vi "connect.vi"(0 "Network Manager IP Address or Hostname":string, 1 "Identity":T1 {"type" items=["Client", "Service"]}, 5 "Network Manager port":u16=1875, 9 "timeout ms":i32=10000, 11 "error in":errorcluster, 12 "username":string, 13 "password":string) -> (4 "connection ID":refnum<k5>, 6 "queue out":refnum<queue>, 15 "error out":errorcluster)   [LabVIEW 2010]
uses:
  i3-json-1.0.0-10/JSON Parsing/Get Object Parameter Files/Get Object Parameter - String.vi
  i3-json-1.0.0-10/i3-json.lvlib
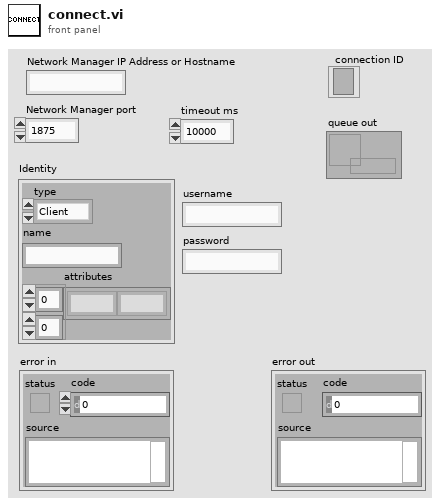
[diagram p1: front panel]
types:
  T1 = cluster{"type":u16, "name":string, "attributes":string[][]}
  T2 = enum16{"Standard", "Buffered", "CRLF", "Immediate"}
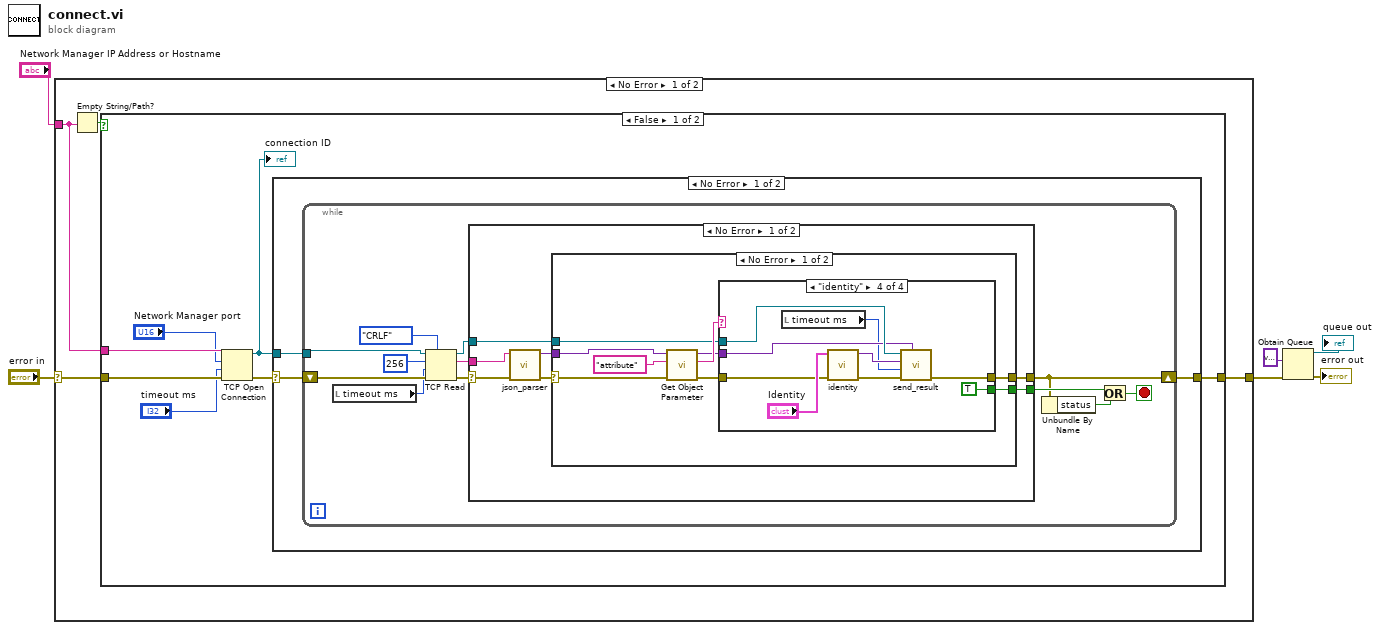
[diagram p0: block diagram]
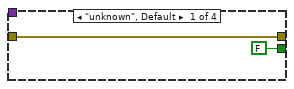
[diagram p2: hidden frame]
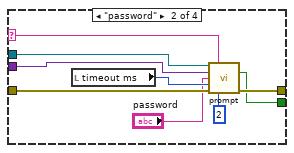
[diagram p3: hidden frame]
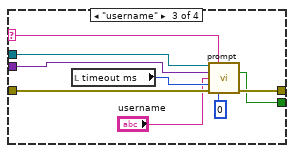
[diagram p4: hidden frame]
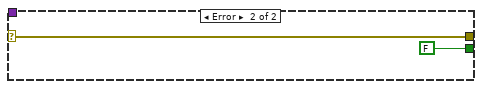
[diagram p5: hidden frame]
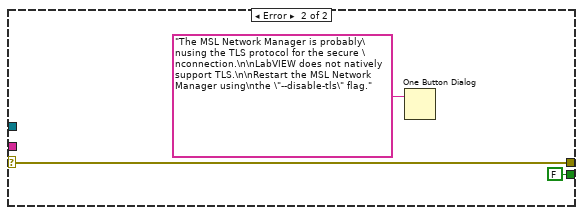
[diagram p6: hidden frame]
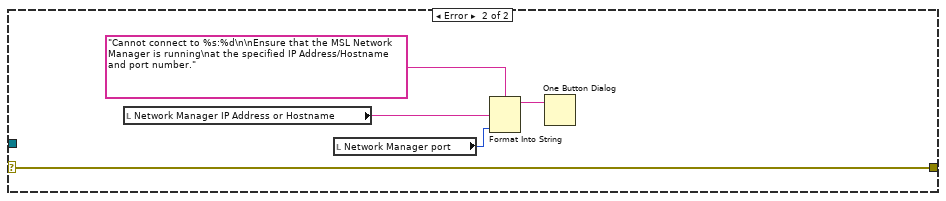
[diagram p7: hidden frame]
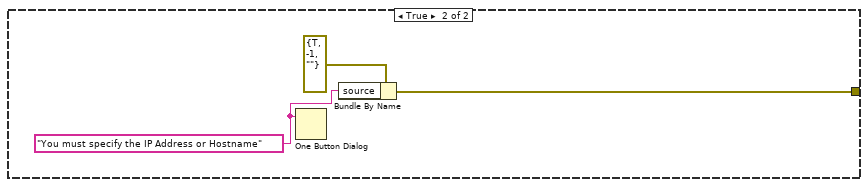
[diagram p8: hidden frame]
diagram:
  n1 = case shown="No Error" "error in" {
    selector: "error in" -> [w8 w91]
    tunnel: [w9 w91] -> w4
    tunnel: "Network Manager IP Address or Hostname" -> [w7 _]
    frame No Error {
      n2 = Empty String/Path?(string/path=w7) -> (empty?=w10:bool)
      n3 = case shown="False" w10 {
        tunnel: [w16 w88] -> w9
        tunnel: w8 -> [w15 _]
        tunnel: w7 -> [w13 _]
        frame False {
          n4 = TCP Open Connection(address=w13, remote port or service name="Network Manager port", timeout ms (60000)="timeout ms", error in (no error)=w15) -> (connection ID=w14:refnum<k5>, error out=w17:errorcluster)  [unwired: 1 in]
          "connection ID" <- w14
          n5 = case shown="No Error" w17 {
            selector: w17 -> [w20 w85]
            tunnel: [w19 w85] -> w16
            tunnel: w14 -> [w18 _]
            frame No Error {
              n6 = while {
                shift-right: [w22] -> w19
                shift-left: w20 -> [w32]
                tunnel: w18 -> [w26]
                stop <- w23 stop-if-true
                n7 = local read "timeout ms"() -> (w25:i32)
                n8 = TCP Read(connection ID=w26, bytes to read=256 ("32bit integer"), error in (no error)=w32, 7:T2."CRLF" ("mode (standard)"), 9:w25) -> (connection ID out=w27:refnum<k5>, data out=w30:string, error out=w28:errorcluster)
                n9 = case shown="No Error" w28 {
                  selector: w28 -> [w39 w81]
                  tunnel: w30 -> [w33 _]
                  tunnel: [w38 w81] -> w22
                  tunnel: w27 -> [w36 _]
                  tunnel: [w35 FALSE] -> w24
                  frame No Error {
                    n10 = call "json_parser.vi"("error in"=w39, "JSON String"=w33) -> ("error out"=w34:errorcluster, "JSON Tree Out Passthrough"=w37:variant)  [unwired: 8 in]
                    n11 = case shown="No Error" w34 {
                      selector: w34 -> [w40 w79]
                      tunnel: [w48 w79] -> w38
                      tunnel: w37 -> [w46 _]
                      tunnel: w36 -> [w43 _]
                      tunnel: [w41 FALSE] -> w35
                      frame No Error {
                        n12 = call-poly "Get Object Parameter.vi"("error in (no error)"=w40, "Parameter Name"="attribute" ("name"), "JSON Tree In (JSON Object)"=w46) -> ("error out"=w45:errorcluster, "String Value"=w44:string, "JSON Tree Out Passthrough"=w42:variant)  [unwired: 5 in, 1 out]
                        n13 = case shown="\"identity\"" w44 {
                          selector: w44 -> [_ w57 w62 _]
                          tunnel: w45 -> [w50 w54 w65 w76]
                          tunnel: [w50 w53 w64 w73] -> w48
                          tunnel: w43 -> [_ w56 w68 w75]
                          tunnel: w42 -> [_ w55 w67 w72]
                          tunnel: [FALSE w52 w63 TRUE] -> w41
                          frame "unknown", Default {
                          }
                          frame "password" {
                            n14 = local read "timeout ms"() -> (w59:i32)
                            n15 = call "prompt.vi"("connection ID"=w56, "type"=w57, "JSON Tree In (JSON Object)"=w55, "default value"="password", "timeout ms"=w59, "error in"=w54, "Display Style"=u32 2) -> ("cancelled?"=w52:bool, "error out"=w53:errorcluster)  [unwired: 6 in, 1 out]
                          }
                          frame "username" {
                            n16 = local read "timeout ms"() -> (w66:i32)
                            n17 = call "prompt.vi"("connection ID"=w68, "type"=w62, "JSON Tree In (JSON Object)"=w67, "default value"="username", "timeout ms"=w66, "error in"=w65, "Display Style"=u32 0) -> ("cancelled?"=w63:bool, "error out"=w64:errorcluster)  [unwired: 6 in, 1 out]
                          }
                          frame "identity" {
                            n18 = local read "timeout ms"() -> (w69:i32)
                            n19 = call "identity.vi"("error in"=w76, "Identity"="Identity") -> ("error out"=w74:errorcluster, "JSON Tree out (JSON Object)"=w71:variant)  [unwired: 8 in]
                            n20 = call "send_result.vi"("JSON Tree In (JSON Object)"=w72, "error in"=w74, "timeout ms"=w69, "result"=w71, "connection ID"=w75) -> ("error out"=w73:errorcluster)  [unwired: 3 in, 3 out]
                          }
                        }
                      }
                      frame Error {
                      }
                    }
                  }
                  frame Error {
                    n21 = One Button Dialog(message="The MSL Network Manager is probably\nusing the TLS protocol for the secure \nconnection.\n\nLabVIEW does not natively support TLS.\n\nRestart the MSL Network Manager using\nthe \"--disable-tls\" flag.") -> ()  [unwired: 1 in, 1 out]
                  }
                }
                n22 = Unbundle By Name(w22) -> ("status"=w21:bool)
                n23 = Or(x=w24, y=w21) -> (x .or. y?=w23:bool)
              }
            }
            frame Error {
              n24 = local read "Network Manager IP Address or Hostname"() -> (w84:string)
              n25 = local read "Network Manager port"() -> (w83:u16)
              n26 = Format Into String(format string="Cannot connect to %s:%d\n\nEnsure that the MSL Network Manager is running\nat the specified IP Address/Hostname and port number.", w84, w83) -> (resulting string=w86:string)  [unwired: 2 in, 1 out]
              n27 = One Button Dialog(message=w86) -> ()  [unwired: 1 in, 1 out]
            }
          }
        }
        frame True {
          w90 = "You must specify the IP Address or Hostname" ("error source (\" \")")
          n28 = One Button Dialog(message=w90) -> ()  [unwired: 1 in, 1 out]
          n29 = Bundle By Name(cluster=errorcluster {"status"=TRUE, "code"=-1, "source"=""} ("error out"), "source"=w90) -> (w88:errorcluster)
        }
      }
    }
    frame Error {
    }
  }
  n30 = Obtain Queue(element data type=variant ("JSON Tree"), error in (no error)=w4) -> (queue out=→"queue out":refnum<queue>, error out=→"error out":errorcluster)  [unwired: 3 in, 1 out]
